vi "Get_Sweep_Cycle.vi"(8 "error in (no error)":errorcluster, 11 ".NET Reference in":refnum<k24>) -> (0 "error out":errorcluster, 2 "times out":i32, 3 ".NET Reference out":refnum<k24>)   [LabVIEW 2017]
uses:
  C:/Users/Ssantec_Test/Documents/Instrument_DLL_Sample_Labview_20220902_Ver1.2.2/DLL/x86/InstrumentDLL.dll
  DLL/x86/InstrumentDLL.dll
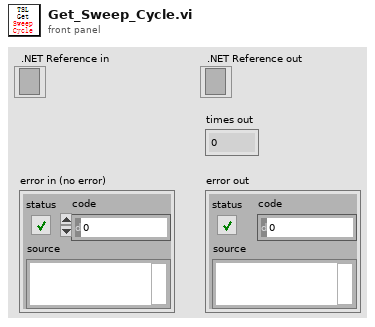
[diagram p1: front panel]
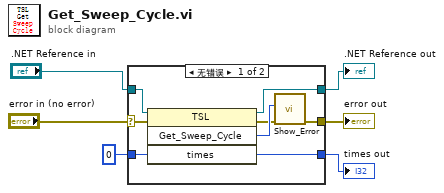
[diagram p0: block diagram]
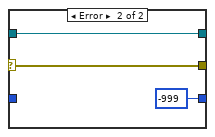
[diagram p2: hidden frame]
diagram:
  n1 = case shown="无错误" "error in (no error)" {
    selector: "error in (no error)" -> [w7 w17]
    tunnel: [w14 -999 ("times")] -> w6
    tunnel: [w8 w17] -> w5
    tunnel: [w13 w16] -> w4
    tunnel: ".NET Reference in" -> [w12 w16]
    tunnel: 0 ("times") -> [w11 _]
    frame No Error {
      n2 = invoke on="调用节点" class="TSL" method="Get_Sweep_Cycle"(reference=w12, error in=w7, "times"=w11) -> (reference out=w13:refnum<k24>, error out=w9:errorcluster, "Get_Sweep_Cycle"=w10:i32, "times"=w14:i32)  [unwired: 1 in]
      n3 = call "Show_Error.vi"("error in (no error)"=w9, "Error"=w10) -> ("error out"=w8:errorcluster)  [unwired: 9 in]
    }
    frame Error {
    }
  }
  "times out" <- w6
  "error out" <- w5
  ".NET Reference out" <- w4
